vi "Untitled 2.vi"() -> ()   [LabVIEW 2009]
panel:
  out "Image (IMAQ)":T1(plugin-control)
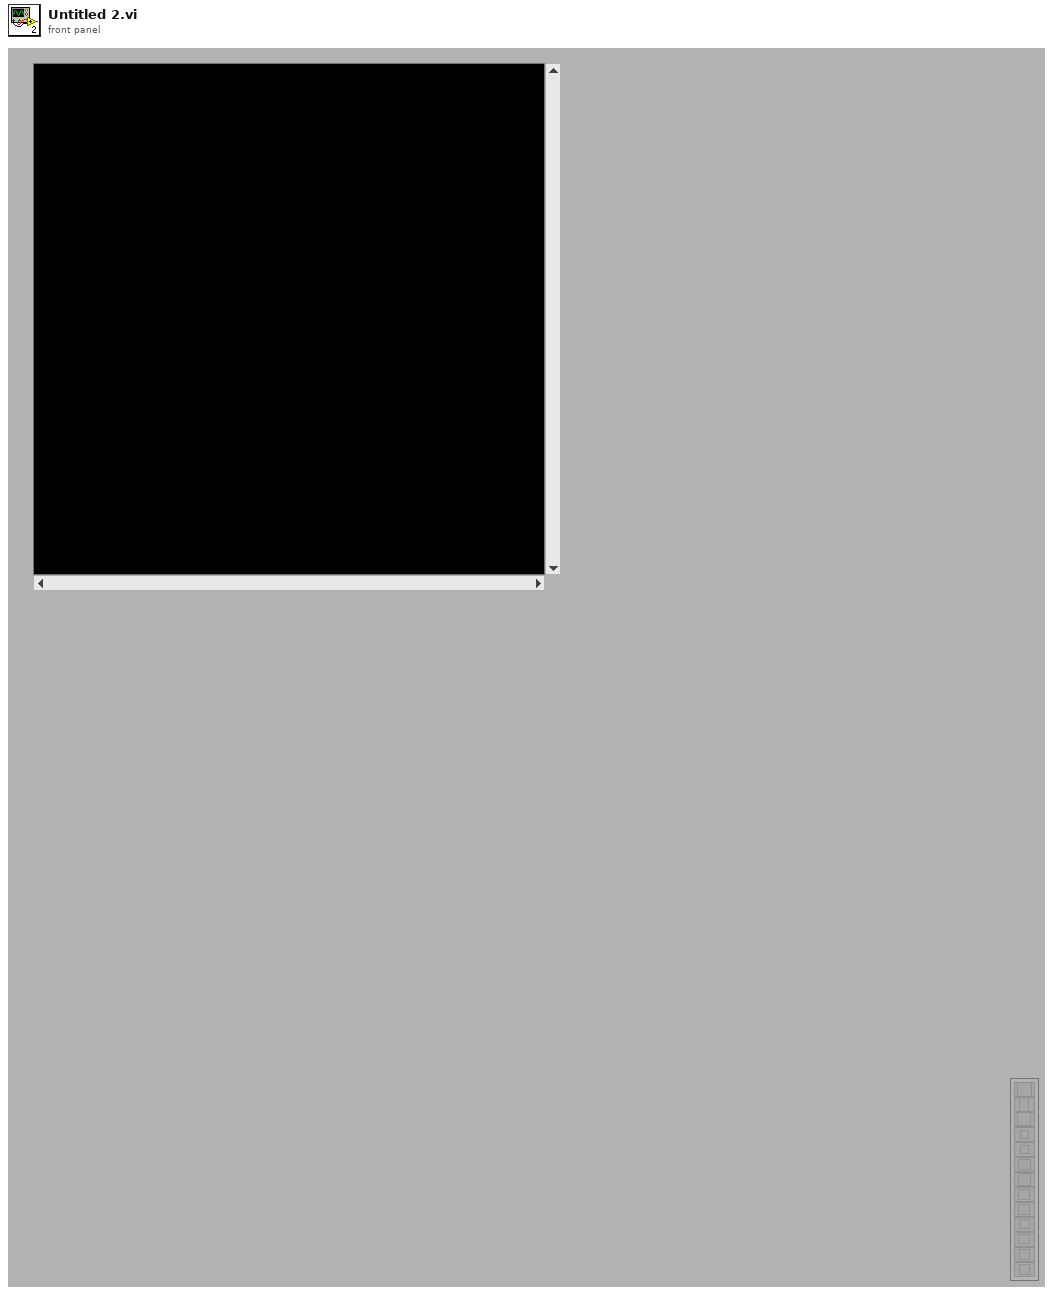
[diagram p1: front panel]
types:
  T1 = typedef "IMAQ Image.ctl" = refnum<image>
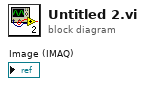
[diagram p0: block diagram]
diagram:
